vi "Field_C open msg.vi"(8 "error in (no error) 2":errorcluster, 9 "timeout ms (2500)":i32=1000, 10 "Connected":bool, 11 "Queue in":T1) -> (0 "error out 2":errorcluster, 2 "Data":variant, 3 "Command":T2, 4 "timed out?":bool, 5 "Unread":i32)   [LabVIEW 2024, in "Magnet module.lvlib"]
doc: "Reads message recived by magnet module. If timeout expire, result will be \"ignore\" command."
uses:
  Magnet module.lvlib
  ctl/Magnet Orders.ctl
  Messenger service/Data types/Mailbox address.ctl
  ctl/MSG to magnet.ctl
  ctl/Tmp_M commands.ctl
  Messenger service/MessengerLib.lvlib
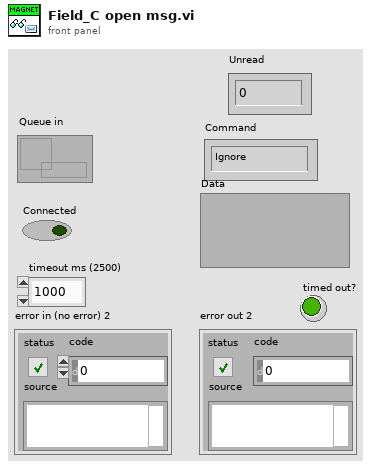
[diagram p1: front panel]
types:
  T1 = typedef "MessengerLib.lvlib/Mailbox address.ctl" = refnum<queue>
  T2 = typedef "Magnet module.lvlib/Magnet Orders.ctl" = enum16{"Ignore", "Connect", "Update", "Switch mode", "Set field", "Stop ramping", "Equalize output", "Zero output", "Flip polarity", "Blackout", "Set timer", "Eval temperatures", "Disconnect"}
  T3 = typedef "Magnet module.lvlib/MSG to magnet.ctl" = cluster{"Command":T2, "Data":variant}
  T4 = typedef "Magnet module.lvlib/Tmp_M commands.ctl" = enum16{"Ignore", "Log", "Connect", "Set timeout", "Update", "Disconnect", "End"}
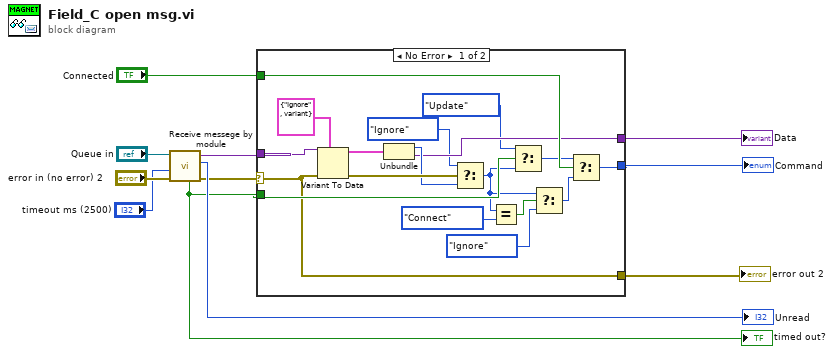
[diagram p0: block diagram]
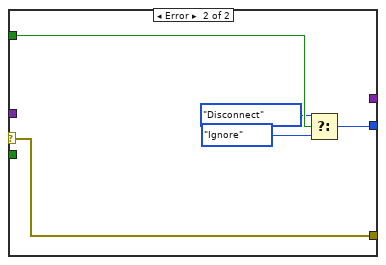
[diagram p2: hidden frame]
diagram:
  n1 = call "Receive messege by module.vi"("error in (no error)"="error in (no error) 2", "timeout in ms (-1)"="timeout ms (2500)", "Module mailbox"="Queue in") -> ("error out"=w6:errorcluster, "Unread"=→"Unread":i32, "Data"=w5:variant, "timed out?"=w7:bool)  [unwired: 4 in, 1 out]
  "timed out?" <- w7
  n2 = case shown="No Error" w6 {
    selector: w6 -> [w20 w34]
    tunnel: w7 -> [w28 _]
    tunnel: [w20 w34] -> w9
    tunnel: "Connected" -> [w29 w31]
    tunnel: w5 -> [w24 _]
    tunnel: [w21 w32] -> w10
    tunnel: [w17 _] -> w8
    frame No Error {
      n3 = Variant To Data(error in=w20, type=T3 {"Command"=enum."Ignore", "Data"=variant(enum16{"Ramping", "Perzistant"} enum."Ramping")} ("MSG to magnet"), Variant=w24) -> (data=w22:T3, error out=w23:errorcluster)
      n4 = Unbundle(w22) -> ("Command"=w19:T2, "Data"=w17:variant)
      n5 = Select(t=Magnet_Orders."Ignore" ("Order"), s=w23, f=w19) -> (s? t:f=w18:T2)
      n6 = Equal?(x=w18, y=Magnet_Orders."Connect" ("Order")) -> (x = y?=w26:bool)
      n7 = Select(t=Magnet_Orders."Update" ("Order"), s=w28, f=w18) -> (s? t:f=w27:T2)
      n8 = Select(t=w18, s=w26, f=Magnet_Orders."Ignore" ("Order")) -> (s? t:f=w25:T2)
      n9 = Select(t=w27, s=w29, f=w25) -> (s? t:f=w21:T2)
    }
    frame Error {
      n10 = Select(t=Tmp_M_commands."Disconnect", s=w31, f=Tmp_M_commands."Ignore" ("Command")) -> (s? t:f=w32:T4)
    }
  }
  "error out 2" <- w9
  "Data" <- w8
  "Command" <- w10
